vi "Switch_Static Dig Path Gen Configure and Generate.vi"(0 "Switch Handle In":refnum<k15>, 5 "Terminal and State Settings":T2={"Connect/Disconnect"=TRUE, "Channel 1"="", "Channel 2"=""}, 11 "error in":errorcluster, 13 "Maximum Wait for Debouce Time":i32=5000) -> (4 "Switch Handle Out":refnum<k15>, 6 "Path Status":T1=1 items=["Other", "Path Available", "Path Exists", "Path Unsupported", "Resource in Use", "Source Conflict", "Channel Not Available"], 15 "error out":errorcluster)   [LabVIEW 2021, in "Switch_Static Digital Path Generation.lvlib"]
doc: "Connects or disconnects a switch path between two specified channels on the NI Switch device from a boolean input. Multiplexers or individual relay switches can be controlled. Enables change of the default value for the maximum length of time to wait for all relays in the switch module to activate or deactivate. Indicates whether a path was valid before applying the Connect/Disconnect action."
uses:
  Switch_Static Digital Path Generation.lvlib
  Typedefs/Terminal and State Settings.ctl
  Typedefs/Path Status.ctl
  <instrlib>/niSwitch/niSwitch.llb/niSwitch Disconnect Channels (Single).vi
  <instrlib>/niSwitch/niSwitch.llb/niSwitch Connect Channels (Single).vi
panel:
  # "Inputs"
  # "Outputs"
  # "Timing Settings"
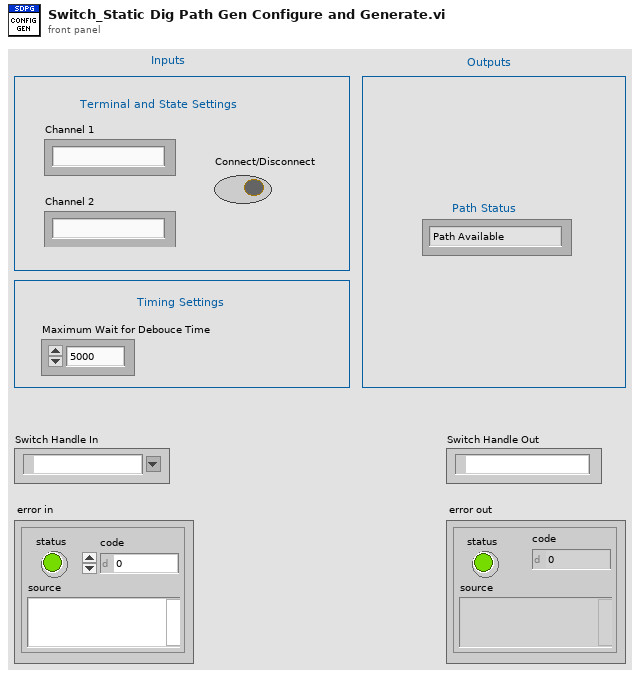
[diagram p1: front panel]
types:
  T1 = typedef "Switch_Static Digital Path Generation.lvlib/Path Status.ctl" = i32
  T2 = typedef "Switch_Static Digital Path Generation.lvlib/Terminal and State Settings.ctl" = cluster{"Connect/Disconnect":bool, "Channel 1":string, "Channel 2":string}
  T3 = typedef "niSwitch Path Capability.ctl" = i32
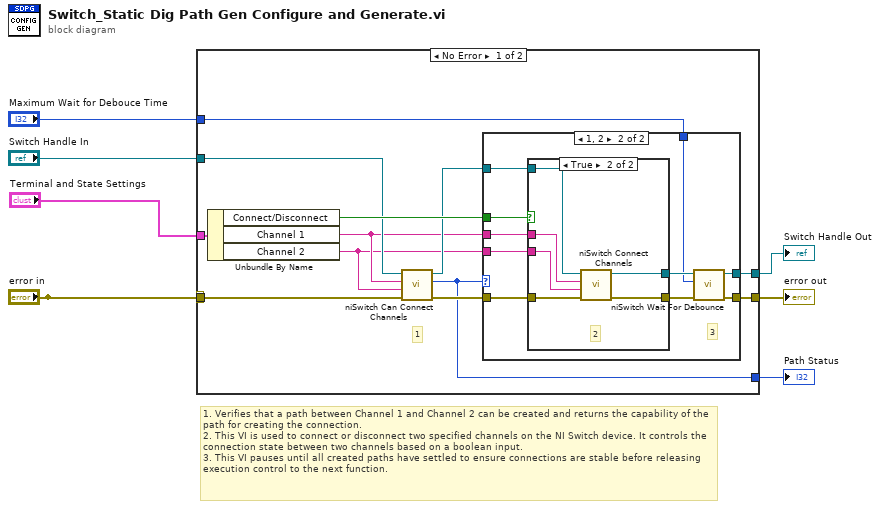
[diagram p0: block diagram]
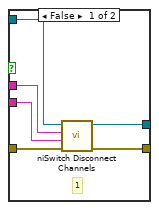
[diagram p3: hidden frame]
diagram:
  # "1. Verifies that a path between Channel 1 and Channel 2 can be created and returns the capability of the path for creating the connection.\n2. This VI is used to connect or disconnect two specified channels on the NI Switch device. It controls the connection state between two channels based on a boolean input.\n3. This VI pauses until all created paths have settled to ensure connections are stable before releasing execution control to the next function."
  n1 = case shown="No Error" "error in" {
    selector: "error in" -> [_ w45]
    tunnel: "Maximum Wait for Debouce Time" -> [w19 _]
    tunnel: [w18 w44] -> w6
    tunnel: "Terminal and State Settings" -> [w17 _]
    tunnel: [w15 w45] -> w4
    tunnel: "Switch Handle In" -> [w14 w44]
    tunnel: "error in" -> [w10 _]
    tunnel: [w8 _] -> w1
    frame No Error {
      # "1"
      n2 = Unbundle By Name(w17) -> ("Connect/Disconnect"=w16:bool, "Channel 1"=w12:string, "Channel 2"=w11:string)
      n3 = call <instrlib>:"niSwitch Can Connect Channels.vi"("error in (no error)"=w10, "channel 2"=w11, "channel 1"=w12, "instrument handle"=w14) -> ("error out"=w9:errorcluster, "path capability"=w8:T3, "instrument handle out"=w13:refnum<k15>)  [unwired: 5 in]
      n4 = case shown="1, 2" w8 {
        tunnel: w19 -> [_ w29]
        tunnel: [w20 w28] -> w18
        tunnel: w16 -> [_ w27]
        tunnel: [w21 w26] -> w15
        tunnel: w13 -> [w20 w25]
        tunnel: w12 -> [_ w24]
        tunnel: w11 -> [_ w23]
        tunnel: w9 -> [w21 w22]
        frame 0, Default {
        }
        frame 1, 2 {
          # "3"
          n5 = case shown="True" w27 {
            tunnel: w25 -> [w36 w43]
            tunnel: [w35 w42] -> w31
            tunnel: w22 -> [w37 w41]
            tunnel: [w34 w40] -> w30
            tunnel: w24 -> [w33 w39]
            tunnel: w23 -> [w32 w38]
            frame False {
              # "1"
              n6 = call-poly <instrlib>:"niSwitch Disconnect Channels.vi"("error in (no error)"=w37, "channel 2"=w32, "channel 1"=w33, "instrument handle"=w36) -> ("error out"=w34:errorcluster, "instrument handle out"=w35:refnum<k15>)  [unwired: 6 in]
            }
            frame True {
              # "2"
              n7 = call-poly <instrlib>:"niSwitch Connect Channels.vi"("error in (no error)"=w41, "channel 2"=w38, "channel 1"=w39, "instrument handle"=w43) -> ("error out"=w40:errorcluster, "instrument handle out"=w42:refnum<k15>)  [unwired: 6 in]
            }
          }
          n8 = call <instrlib>:"niSwitch Wait For Debounce.vi"("error in (no error)"=w30, "maximum time (5000 ms)"=w29, "instrument handle"=w31) -> ("error out"=w26:errorcluster, "instrument handle out"=w28:refnum<k15>)  [unwired: 7 out]
        }
      }
    }
    frame Error {
    }
  }
  "Switch Handle Out" <- w6
  "error out" <- w4
  "Path Status" <- w1
